vi "RT 16 bit ADC DAC_KA.vi"() -> ()   [LabVIEW 2018]
doc: "The myRIO Custom FPGA Project template acquires button data from the onboard button and displays the button value on a Boolean indicator. The SYS.RDY indicator shows the FPGA status."
uses:
  <vilib>/rvi/interface/nirviCloseFPGA/nirviCloseFPGA.xnode
  <vilib>/rvi/interface/nirviOpenFPGA/nirviOpenFPGA.xnode
  <vilib>/rvi/interface/nirviReadWriteControl/nirviReadWriteControl.xnode
  NiFpgaLv.dll
  <vilib>/Utility/error.llb/Error Cluster From Error Code.vi
  <vilib>/rvi/interface/Simulation/niFpgaSimulationCallBeginRW.vi
  <vilib>/rvi/errors/niLvFpgaAdjustHostInterfaceError.vi
  <vilib>/FPGAPlugInAG/Dynamic/niLvFpga_Close_Dynamic.vi
  FPGA Bitfiles/ASPE2019StudentC_FPGATarget_FPGASPI_ZCDGpJzZuc4.lvbitx
  16Bit_ADC_DAC/FPGA_SPI.vi
  <vilib>/FPGAPlugInAG/myRIO-1900/niLvFpga_Open_myRIO-1900.vi
  <vilib>/rvi/interface/common/dynamic/niFpgaDynamicAddResources.vi
panel:
  in  "CH1":bool[](array[boolean])=[FALSE, FALSE, TRUE, FALSE, FALSE, TRUE, FALSE, FALSE, FALSE, FALSE, FALSE, FALSE, FALSE, FALSE, FALSE, FALSE]
  in  "CH3":bool[](array[boolean])=[FALSE, FALSE, FALSE, TRUE, FALSE, TRUE, FALSE, FALSE, FALSE, FALSE, FALSE, FALSE, FALSE, FALSE, FALSE, FALSE]
  in  "CH2":bool[](array[boolean])=[FALSE, FALSE, FALSE, FALSE, FALSE, TRUE, FALSE, FALSE, FALSE, FALSE, FALSE, FALSE, FALSE, FALSE, FALSE, FALSE]
  out "avg. loop rate (kHz)":dbl
  in  "time delay":u32=1
  out "sense (Force mode)":dbl(graph)
  out "EMF (Velocity mode)":dbl(graph)
  out "Cap probe":dbl(graph)=0.00030517112470818
  in  "Amplitude":dbl=1.0 format="%0.3p"
  in  "samples per cycle":u32=1000
  in  "stop":bool
  in  "Color Box":u32(colorbox)
  in  "?":u32(colorbox)
  # "Force mode"
  # "Velocity mode"
  # "DAC"
  # "ADC"
  # "when you write to channel 2 of ADC, \nyou read previous channel, ch 1 to which cap probe is connected to.  \nRef:Table 1,2: ADC LTC1859"
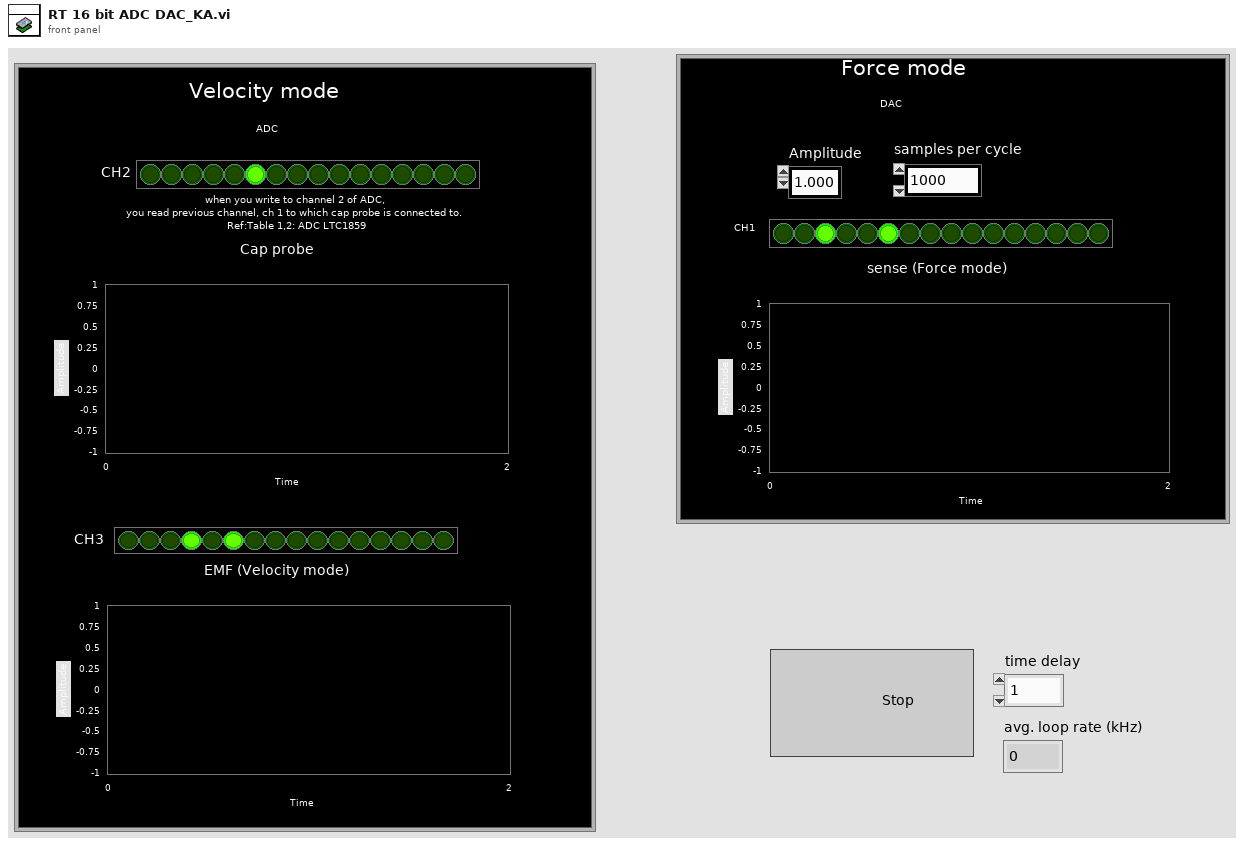
[diagram p1: front panel]
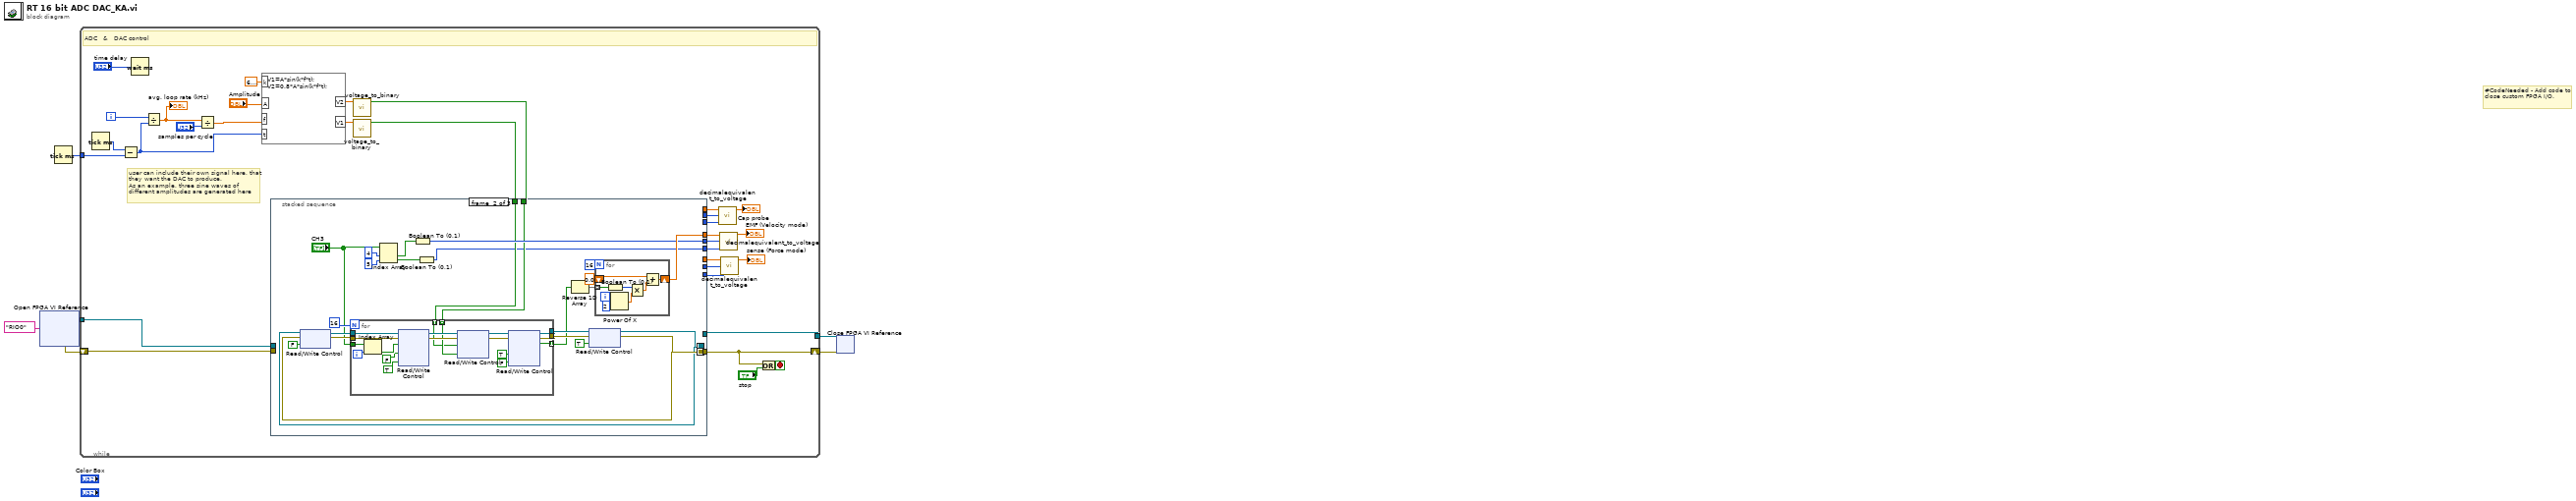
[diagram p0: block diagram]
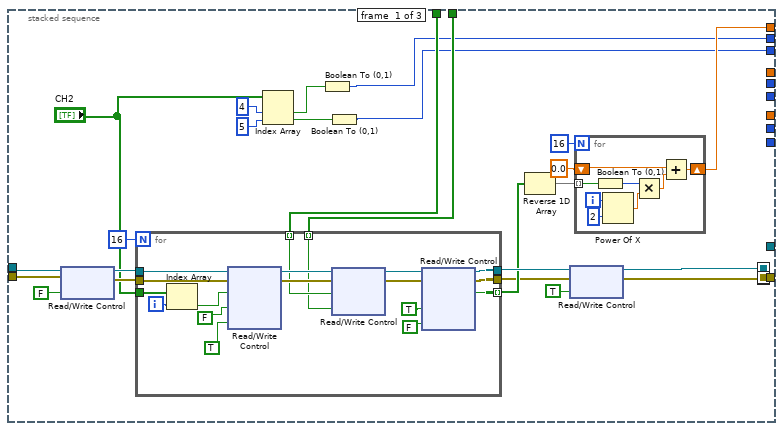
[diagram p2: hidden frame]
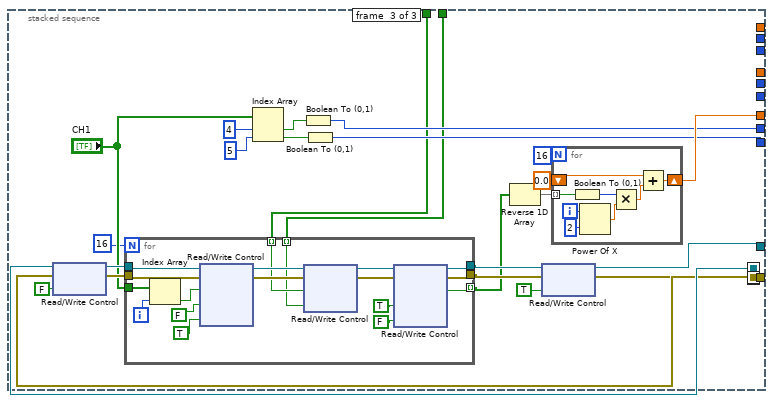
[diagram p3: hidden frame]
diagram:
  # "#CodeNeeded - Add code to close custom FPGA I/O."
  n1 = xnode "Open FPGA VI Reference"("resource name"=tag "RIO0") -> ("FPGA VI Reference Out"=w5:refnum<k20>, "error out"=w4:errorcluster)  [unwired: 1 in]
  n2 = Tick Count (ms)() -> (millisecond timer value=w2:u32)
  n3 = while {
    shift-right: [w25] -> w6
    shift-left: w4 -> [w30]
    tunnel: w2 -> [w36]
    tunnel: w5 -> [w31]
    tunnel: [w26] -> w1
    i -> [w32]
    stop <- w37 stop-if-true
    # "user can include their own signal here, that \nthey want the DAC to produce.\nAs an example, three sine waves of \ndifferent amplitudes are generated here"
    # "ADC   &   DAC control"
    n4 = Tick Count (ms)() -> (millisecond timer value=w34:u32)
    n5 = Subtract(x=w34, y=w36) -> (x-y=w23:u32)
    n6 = Wait (ms)(milliseconds to wait="time delay") -> ()  [unwired: 1 out]
    n7 = Divide(x=w32, y=w23) -> (x/y=w33:dbl)
    "avg. loop rate (kHz)" <- w33
    n8 = Divide(x=w33, y="samples per cycle") -> (x/y=w27:dbl)
    n9 = formula code="V1=A*sin(k*f*t);\nV2=0.8*A*sin(k*f*t);"("t"=w23, "f"=w27, "A"="Amplitude", "k"=6.283185307179586 ("input variable")) -> ("V1"=w13:dbl, "V2"=w11:dbl)
    n10 = call "voltage_to_binary.vi"("voltage"=w11) -> ("binary"=w10:bool[])  [unwired: 10 in]
    n11 = call "voltage_to_binary.vi"("voltage"=w13) -> ("binary"=w12:bool[])  [unwired: 10 in]
    n12 = stacked-sequence {
      seq-local: [w58 _ _] -> [_ w108 _]
      seq-local: [w57 _ _] -> [_ w107 _]
      seq-local: [_ w110 _] -> [_ _ w161]
      seq-local: [_ w109 _] -> [_ _ w160]
      tunnel: [w56 _ _] -> w22
      tunnel: [_ w106 _] -> w21
      tunnel: [_ _ w159] -> w26
      tunnel: [_ _ w158] -> w25
      tunnel: [_ _ w157] -> w20
      tunnel: w31 -> [w55 _ _]
      tunnel: w30 -> [w54 _ _]
      tunnel: [w41 _ _] -> w19
      tunnel: [w40 _ _] -> w16
      tunnel: [_ w101 _] -> w18
      tunnel: [_ w93 _] -> w15
      tunnel: [_ _ w156] -> w17
      tunnel: [_ _ w155] -> w14
      tunnel: w12 -> [w51 w95 w147]
      tunnel: w10 -> [w46 w94 w144]
      frame #0 {
        n13 = xnode "Read/Write Control"("FPGA VI Reference In"=w55, "error in"=w54, "CS"=FALSE) -> ("FPGA VI Reference Out"=w53:refnum<k20>, "error out"=w52:errorcluster)
        n14 = for {
          N: 16 -> [_]
          tunnel: w53 -> [w81]
          tunnel: w52 -> [w80]
          tunnel: [w79] -> w49 mode=indexing
          tunnel: [w78] -> w50
          tunnel: [w77] -> w48
          tunnel: "CH2" -> [w74]
          tunnel: w51 -> [w67] mode=indexing
          tunnel: w46 -> [w66] mode=indexing
          i -> [w76]
          n15 = Index Array(array=w74, index=w76) -> (element=w75:bool)
          n16 = xnode "Read/Write Control"("FPGA VI Reference In"=w81, "error in"=w80, "MOSI1"=w75, "CLK2"=FALSE ("CLK"), "CLK1"=TRUE ("CLK")) -> ("FPGA VI Reference Out"=w71:refnum<k20>, "error out"=w70:errorcluster)
          n17 = xnode "Read/Write Control"("FPGA VI Reference In"=w71, "error in"=w70, "MOSI2"=w67, "MOSI3"=w66) -> ("FPGA VI Reference Out"=w69:refnum<k20>, "error out"=w68:errorcluster)
          n18 = xnode "Read/Write Control"("FPGA VI Reference In"=w69, "error in"=w68, "CLK2"=TRUE, "CLK1"=FALSE) -> ("FPGA VI Reference Out"=w78:refnum<k20>, "error out"=w77:errorcluster, "MISO1"=w79:bool)
        }
        n19 = Index Array(array="CH2", index #1=4 ("index"), index #2=5 ("index")) -> (element #1=w43:bool, element #2=w42:bool)
        n20 = Boolean To (0,1)(Boolean=w43) -> (0, 1=w41:i16)
        n21 = Boolean To (0,1)(Boolean=w42) -> (0, 1=w40:i16)
        n22 = Reverse 1D Array(array=w49) -> (reversed array=w61:bool[])
        n23 = xnode "Read/Write Control"("FPGA VI Reference In"=w50, "error in"=w48, "CS"=TRUE) -> ("FPGA VI Reference Out"=w58:refnum<k20>, "error out"=w57:errorcluster)
        n24 = for {
          N: 16 -> [_]
          shift-right: [w82] -> w56
          shift-left: 0.0 -> [w88]
          tunnel: w61 -> [w83] mode=indexing
          i -> [w84]
          n25 = Boolean To (0,1)(Boolean=w83) -> (0, 1=w89:i16)
          n26 = Power Of X(1:2 ("y"), 2:w84) -> (0:w86:dbl)
          n27 = Multiply(x=w89, y=w86) -> (x*y=w87:dbl)
          n28 = Add(x=w88, y=w87) -> (x+y=w82:dbl)
        }
      }
      frame #1 {
        n29 = xnode "Read/Write Control"("FPGA VI Reference In"=w108, "error in"=w107, "CS"=FALSE) -> ("FPGA VI Reference Out"=w100:refnum<k20>, "error out"=w99:errorcluster)
        n30 = for {
          N: 16 -> [_]
          tunnel: w100 -> [w123]
          tunnel: w99 -> [w122]
          tunnel: [w116] -> w96 mode=indexing
          tunnel: [w118] -> w98
          tunnel: [w117] -> w97
          tunnel: "CH3" -> [w121]
          tunnel: w95 -> [w119] mode=indexing
          tunnel: w94 -> [w120] mode=indexing
          i -> [w115]
          n31 = Index Array(array=w121, index=w115) -> (element=w132:bool)
          n32 = xnode "Read/Write Control"("FPGA VI Reference In"=w123, "error in"=w122, "MOSI1"=w132, "CLK2"=FALSE ("CLK"), "CLK1"=TRUE ("CLK")) -> ("FPGA VI Reference Out"=w129:refnum<k20>, "error out"=w128:errorcluster)
          n33 = xnode "Read/Write Control"("FPGA VI Reference In"=w129, "error in"=w128, "MOSI2"=w119, "MOSI3"=w120) -> ("FPGA VI Reference Out"=w127:refnum<k20>, "error out"=w126:errorcluster)
          n34 = xnode "Read/Write Control"("FPGA VI Reference In"=w127, "error in"=w126, "CLK2"=TRUE, "CLK1"=FALSE) -> ("FPGA VI Reference Out"=w118:refnum<k20>, "error out"=w117:errorcluster, "MISO1"=w116:bool)
        }
        n35 = Index Array(array="CH3", index #1=4 ("index"), index #2=5 ("index")) -> (element #1=w103:bool, element #2=w102:bool)
        n36 = Boolean To (0,1)(Boolean=w103) -> (0, 1=w101:i16)
        n37 = Boolean To (0,1)(Boolean=w102) -> (0, 1=w93:i16)
        n38 = Reverse 1D Array(array=w96) -> (reversed array=w112:bool[])
        n39 = xnode "Read/Write Control"("FPGA VI Reference In"=w98, "error in"=w97, "CS"=TRUE) -> ("FPGA VI Reference Out"=w110:refnum<k20>, "error out"=w109:errorcluster)
        n40 = for {
          N: 16 -> [_]
          shift-right: [w138] -> w106
          shift-left: 0.0 -> [w139]
          tunnel: w112 -> [w133] mode=indexing
          i -> [w134]
          n41 = Boolean To (0,1)(Boolean=w133) -> (0, 1=w140:i16)
          n42 = Power Of X(1:2 ("y"), 2:w134) -> (0:w136:dbl)
          n43 = Multiply(x=w140, y=w136) -> (x*y=w137:dbl)
          n44 = Add(x=w139, y=w137) -> (x+y=w138:dbl)
        }
      }
      frame #2 {
        n45 = xnode "Read/Write Control"("FPGA VI Reference In"=w161, "error in"=w160, "CS"=FALSE) -> ("FPGA VI Reference Out"=w146:refnum<k20>, "error out"=w145:errorcluster)
        n46 = for {
          N: 16 -> [_]
          tunnel: w146 -> [w174]
          tunnel: w145 -> [w173]
          tunnel: [w168] -> w148 mode=indexing
          tunnel: [w167] -> w150
          tunnel: [w166] -> w149
          tunnel: "CH1" -> [w172]
          tunnel: w147 -> [w170] mode=indexing
          tunnel: w144 -> [w169] mode=indexing
          i -> [w171]
          n47 = Index Array(array=w172, index=w171) -> (element=w183:bool)
          n48 = xnode "Read/Write Control"("FPGA VI Reference In"=w174, "error in"=w173, "MOSI1"=w183, "CLK2"=FALSE ("CLK"), "CLK1"=TRUE ("CLK")) -> ("FPGA VI Reference Out"=w180:refnum<k20>, "error out"=w179:errorcluster)
          n49 = xnode "Read/Write Control"("FPGA VI Reference In"=w180, "error in"=w179, "MOSI2"=w170, "MOSI3"=w169) -> ("FPGA VI Reference Out"=w178:refnum<k20>, "error out"=w177:errorcluster)
          n50 = xnode "Read/Write Control"("FPGA VI Reference In"=w178, "error in"=w177, "CLK2"=TRUE, "CLK1"=FALSE) -> ("FPGA VI Reference Out"=w167:refnum<k20>, "error out"=w166:errorcluster, "MISO1"=w168:bool)
        }
        n51 = Index Array(array="CH1", index #1=4 ("index"), index #2=5 ("index")) -> (element #1=w152:bool, element #2=w151:bool)
        n52 = Boolean To (0,1)(Boolean=w152) -> (0, 1=w156:i16)
        n53 = Boolean To (0,1)(Boolean=w151) -> (0, 1=w155:i16)
        n54 = Reverse 1D Array(array=w148) -> (reversed array=w163:bool[])
        n55 = xnode "Read/Write Control"("FPGA VI Reference In"=w150, "error in"=w149, "CS"=TRUE) -> ("FPGA VI Reference Out"=w159:refnum<k20>, "error out"=w158:errorcluster)
        n56 = for {
          N: 16 -> [_]
          shift-right: [w189] -> w157
          shift-left: 0.0 -> [w190]
          tunnel: w163 -> [w184] mode=indexing
          i -> [w185]
          n57 = Boolean To (0,1)(Boolean=w184) -> (0, 1=w191:i16)
          n58 = Power Of X(1:2 ("y"), 2:w185) -> (0:w187:dbl)
          n59 = Multiply(x=w191, y=w187) -> (x*y=w188:dbl)
          n60 = Add(x=w190, y=w188) -> (x+y=w189:dbl)
        }
      }
    }
    n61 = call "decimalequivalent_to_voltage.vi"("GAIN"=w16, "UNI"=w19, "i"=w22) -> ("V"=→"Cap probe":dbl)  [unwired: 8 in]
    n62 = call "decimalequivalent_to_voltage.vi"("GAIN"=w15, "UNI"=w18, "i"=w21) -> ("V"=→"EMF (Velocity mode)":dbl)  [unwired: 8 in]
    n63 = call "decimalequivalent_to_voltage.vi"("GAIN"=w14, "UNI"=w17, "i"=w20) -> ("V"=→"sense (Force mode)":dbl)  [unwired: 8 in]
    n64 = Or(x=w25, y="stop") -> (x .or. y?=w37:bool)
  }
  n65 = xnode "Close FPGA VI Reference"("FPGA VI Reference In"=w1, "error in"=w6) -> ()  [unwired: 1 out]
